vi "readRegisterS0_8.vi"(8 "error in (no error)":errorcluster, 10 "Offset":u32) -> (0 "error out":errorcluster, 3 "Data 1":u8=255)   [LabVIEW 2015, in "ESLSCDLL.lvlib"]
uses:
  ESLSCDLL.lvlib
  Globals.vi
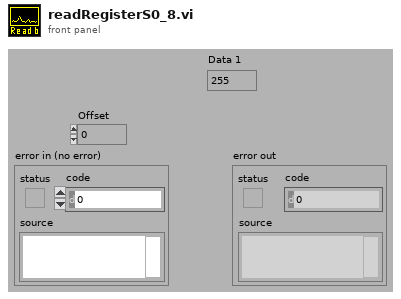
[diagram p1: front panel]
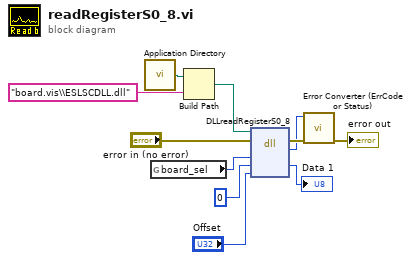
[diagram p0: block diagram]
diagram:
  n1 = call <vilib>:"Application Directory.vi"() -> ("Application Directory"=w5:path)
  n2 = global read "Globals.vi" "board_sel"() -> (w2:u32)
  n3 = Build Path(base path=w5, name or relative path="board.vis\\ESLSCDLL.dll") -> (appended path=w3:path)
  n4 = dll-call lib="C:/ENTW/PCIE/LV64/board.vis/ESLSCDLL.dll" fn="DLLreadRegisterS0_8" ("lwlscdll.dll:DLLReadByteS0")(path in=w3, error in="error in (no error)", "board_sel"=w2, "data"=u8 0, "PortOff"="Offset") -> (error out=w7:errorcluster, "es_status_codes"=w6:i32, "data"=→"Data 1":u8)  [unwired: 3 in, 1 out]
  n5 = call "Error Converter (ErrCode or Status).vi"("error in (no error)"=w7, "error code"=w6) -> ("error out"=→"error out":errorcluster)  [unwired: 9 in]
